vi "LEBITlib.getDNSFQName.vi"() -> (0 "DNSFQName":string)   [LabVIEW 2014, in "LEBITLib.lvlib"]
doc: "REV6250"
uses:
  LEBITLib.lvlib
  kernel32.dll
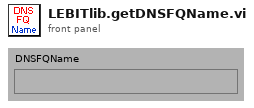
[diagram p1: front panel]
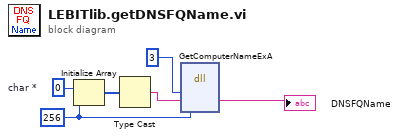
[diagram p0: block diagram]
diagram:
  w4 = 256 ("dimension size")
  w6 = u8 0  # char *
  n1 = Initialize Array(w6, w4) -> (w5:u8[])
  n2 = Type Cast(x=w5) -> (*(type *) &x=w3:string)  [unwired: 1 in]
  n3 = dll-call lib="kernel32.dll" fn="GetComputerNameExA" label="unsigned long GetComputerNameExA(int cnf, CStr lpBuffer, long *nSize);"("cnf"=3, "lpBuffer"=w3, "nSize"=w4) -> ("lpBuffer"=→"DNSFQName":string)  [unwired: 6 in, 2 out]
